vi "4Pi Objective Lock.vi"(7 "Calling VI Ref":refnum<vi>) -> ()   [LabVIEW 2016]
uses:
  Hardware Configuration/Hardware Configuration Controls/Device Type.ctl
  Hardware Configuration/Hardware Configuration Controls/Device Function.ctl
  <vilib>/Utility/miscctls.llb/LVPointTypeDef.ctl
  4Pi Objective Lock Type Defs/4Pi Obj Lock - Actions.ctl
  4Pi Objective Lock Type Defs/4Pi Obj Lock - Notifier Type.ctl
  4Pi Objective Lock Type Defs/4Pi Obj Lock - Lock Settings.ctl
  4Pi Objective Lock Type Defs/4Pi Obj Lock - Camera Settings.ctl
  Device Library/Cameras/Camera Controls/Generic Camera Actions.ctl
  Device Library/Cameras/Camera Controls/Generic Camera ROI.ctl
  <vilib>/addons/control/pid/NI_PID_pid.lvlib
  <vilib>/addons/control/pid/pid.llb/PID (DBL Array).vi
panel:
  in  "Main Tab":T1(tab)
  in  "Update Delay (ms)":i32=10
  in  "D (Derivative)":dbl
  in  "I (Integral)":dbl
  in  "P (Proportional)":dbl=2.0
  in  "Invert Z Axis":bool
  in  "XY Drift Threshold":dbl=0.05
  in  "Abort If Error":bool
  in  "Flip XY Axis":bool
  in  "Invert X Axis":bool
  in  "Invert Y Axis":bool
  in  "Z Stage Move Limit (µm)":dbl=1.0
  in  "Z Drift Threshold":dbl=0.05
  in  "XY Stage Move Limit (µm)":dbl=1.0
  in  "Frame Accumulations":u16=10
  in  "Save Lock Settings":bool
  in  "XY Correction Active":bool=TRUE
  in  "Z Correction Active":bool=TRUE
  in  "Set Camera ROI":bool
  out "Stage Positions":dbl(graph)
  out "Objective Positions":dbl(graph)
  out "X Axis Position (µm)":dbl=1.0
  out "Y Axis Position (µm)":dbl=1.0
  out "Z Axis Position (µm)":dbl=1.0
  out "Measured X Position (px)":dbl=1.0
  out "Measured Y Position (px)":dbl=1.0
  out "Measured Z Position (px)":dbl=1.0
  in  "Start Lock":bool
  out "Error":bool
  in  "Quit":bool
  # "Z Drift Settings"
  # "General Settings"
  # "Camera Setup"
  # "XY Drift Settings"
  # "PID Control Values"
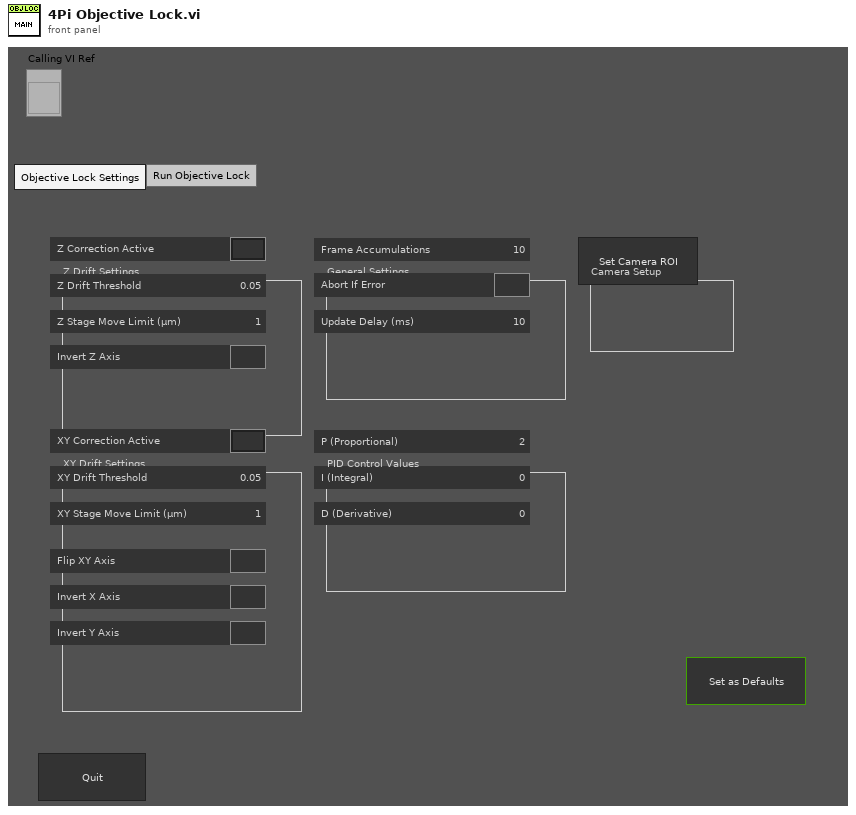
[diagram p1: front panel]
types:
  T1 = enum32{"Objective Lock Settings", "Run Objective Lock"}
  T2 = typedef "4Pi Obj Lock - Camera Settings.ctl" = cluster{"Exposure Time (s)":dbl, "H Offset":u16, "V Offset":u16, "H Width":u16, "V Width":u16}
  T3 = typedef "Device Function.ctl" = enum16{"Primary", "Secondary", "Overview", "Wide Field Drift Correction", "642 nm Excitation", "560 nm Excitation", "546 nm Excitation", "488 nm Excitation", "405 nm Excitation", "Objective Drift Correction", "4Pi Objective Lock", "Objective XY", "Objective Z", "Sample XY", "Sample Coarse Z", "Sample Z", "4Pi Lower", "4Pi Upper", "Adj Cavity", "Line Scanning", "Alert"}
  T4 = typedef "Device Type.ctl" = enum16{"AOTF", "Camera", "Deformable Mirror", "Laser", "Shutter", "Stage", "Waveform", "Email"}
  T5 = typedef "4Pi Obj Lock - Actions.ctl" = enum16{"Idle", "Start Lock", "Get Initial Position", "Get Current Position", "Check Drift", "Move", "Delay", "Abort", "Exit Loop", "Quit"}
  T6 = typedef "4Pi Obj Lock - Lock Settings.ctl" = cluster{"Z Drift Threshold":dbl, "Z Stage Move Limit (µm)":dbl, "XY Drift Threshold":dbl, "XY Stage Move Limit (µm)":dbl, "Frame Accumulations":u16, "Abort If Error":bool, "Flip XY Axis":bool, "Invert X Axis":bool, "Invert Y Axis":bool, "Invert Z Axis":bool, "Z Correction Active":bool, "XY Correction Active":bool, "PID Values":dbl[], "Update Delay (ms)":i32}
  T7 = typedef "4Pi Obj Lock - Notifier Type.ctl" = cluster{"Actions":T5, "Z Drift Threshold":dbl, "Z Stage Move Limit (µm)":dbl, "XY Drift Threshold":dbl, "XY Stage Move Limit (µm)":dbl, "Frame Accumulations":u16, "Abort If Error":bool, "Z Correction Active":bool, "XY Correction Active":bool, "PID Values":dbl[], "Obj Lock Active?":bool, "Update Delay (ms)":i32}
  T8 = enum16{"Always On", "Always Off", "Off While Running"}
  T9 = typedef "LVPointTypeDef.ctl" = cluster{"Horizontal":i16, "Vertical":i16}
  T10 = typedef "Generic Camera Actions.ctl" = enum16{"Status", "Live Preview", "Capture", "Abort", "Set Exposure Time (s)", "Get Exposure Time (s)", "Record Settings", "Set ROI", "Get ROI", "Defect Correction On/Off", "Cooler On/Off", "Fan On/Off", "Quti"}
  T11 = typedef "Generic Camera ROI.ctl" = cluster{"H Offset":u16, "V Offset":u16, "H Width":u16, "V Width":u16}
  T12 = enum32{"Invalid", "Standard", "Closed", "Hidden", "Minimized", "Maximized"}
  T13 = typedef "2D Gaussian - Best Fit Parameters.ctl" = cluster{"Amplitude":dbl, "X Position":dbl, "Y Position":dbl, "X Width":dbl, "Y Width":dbl, "Offset":dbl}
  T14 = cluster{"PID Values[0]":dbl, "PID Values[1]":dbl, "PID Values[2]":dbl}
  T15 = cluster{"PID Values[0]":dbl, "PID Values[1]":dbl, "PID Values[2]":dbl}[]
  T16 = typedef "LVRectTypeDef.ctl" = cluster{"Left":i16, "Top":i16, "Right":i16, "Bottom":i16}
  T17 = typedef "LVBoundsTypeDef.ctl" = cluster{"Width":u32, "Height":u32}
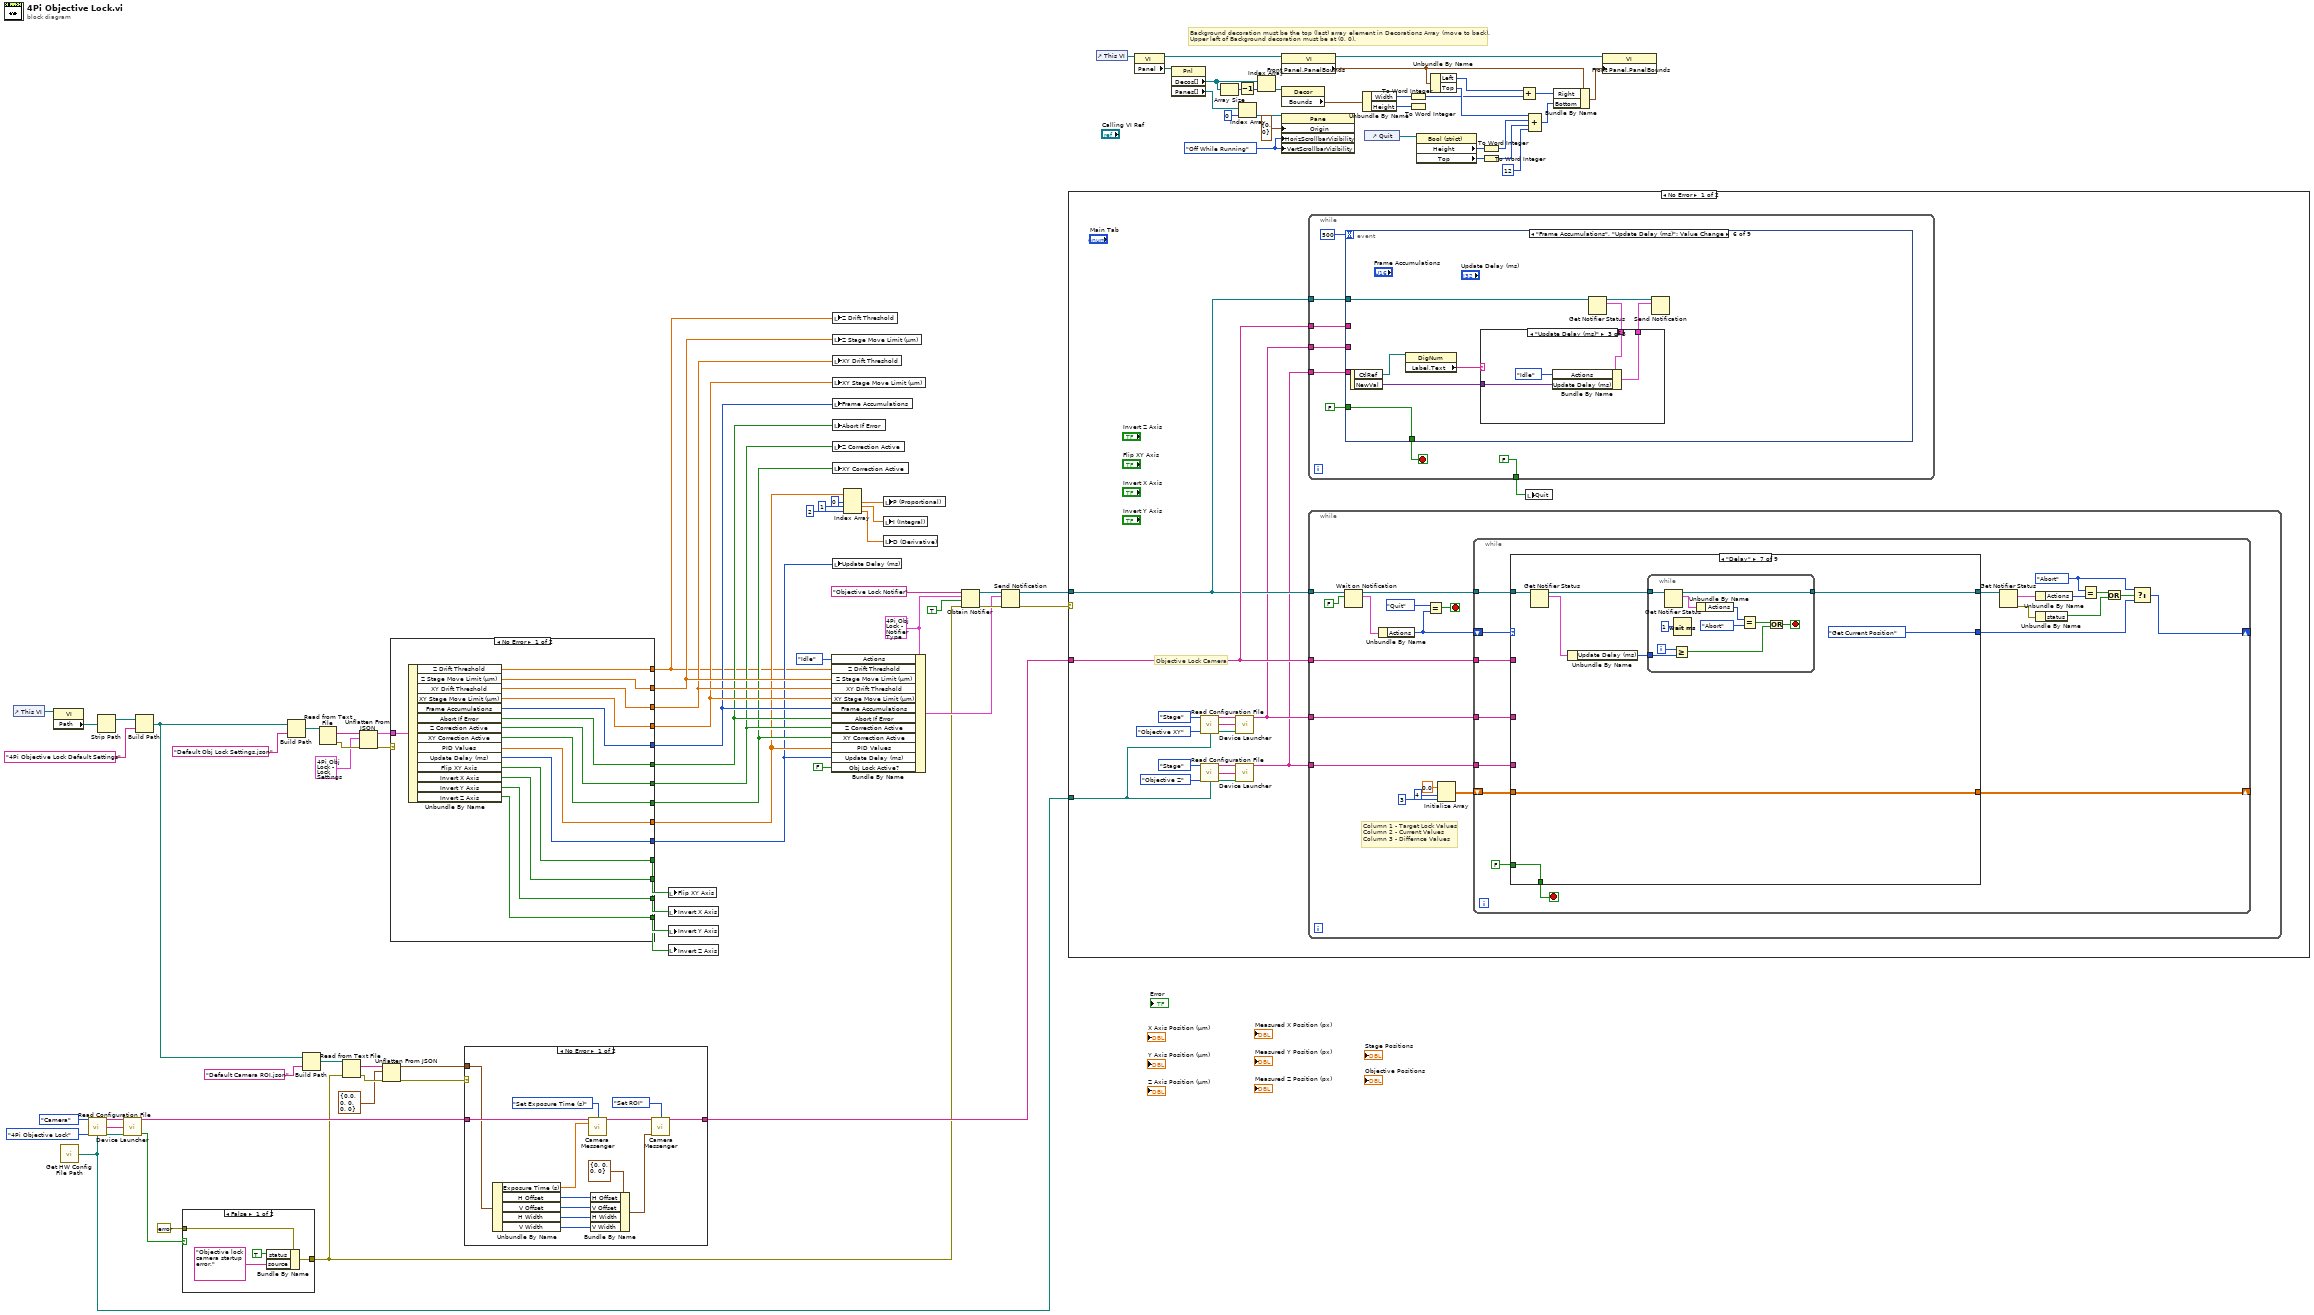
[diagram p0: block diagram]
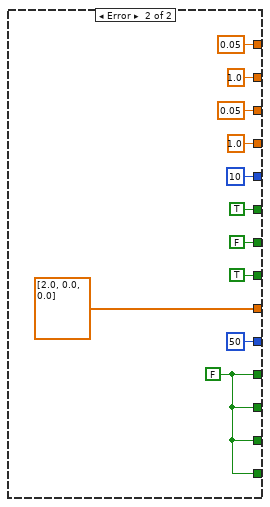
[diagram p4: hidden frame]
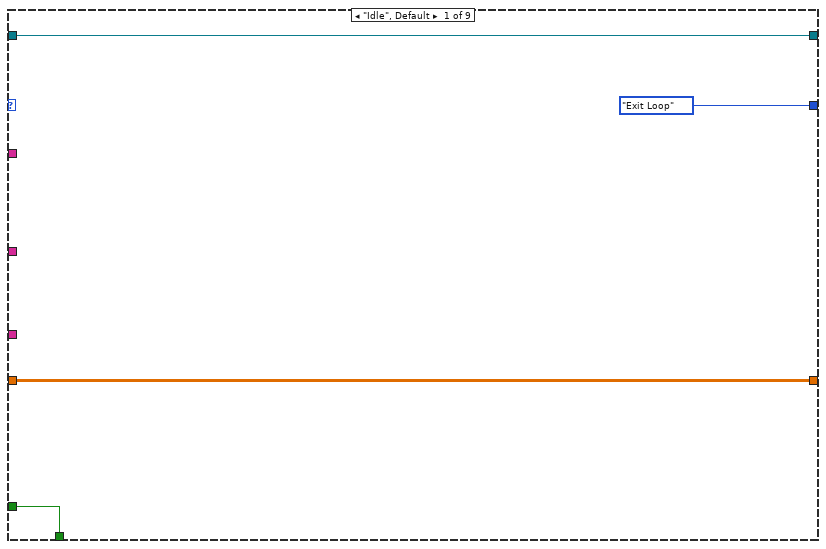
[diagram p5: hidden frame]
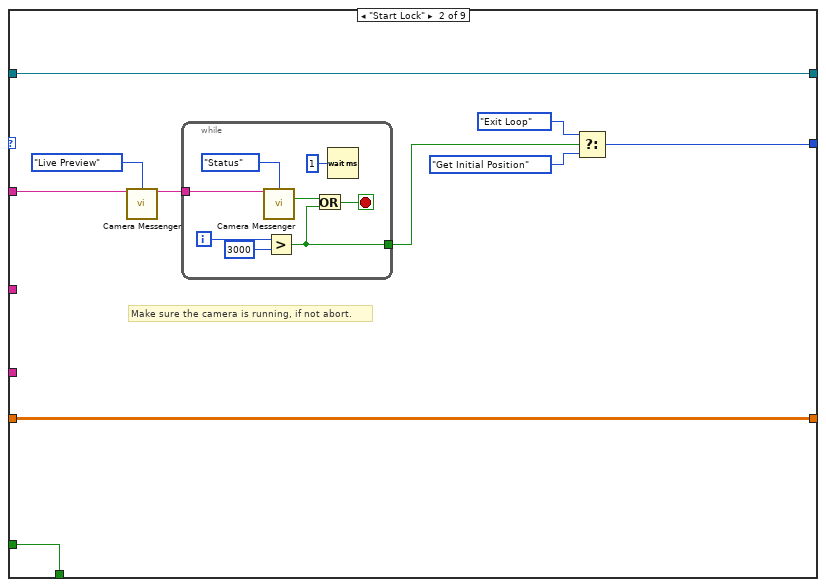
[diagram p6: hidden frame]
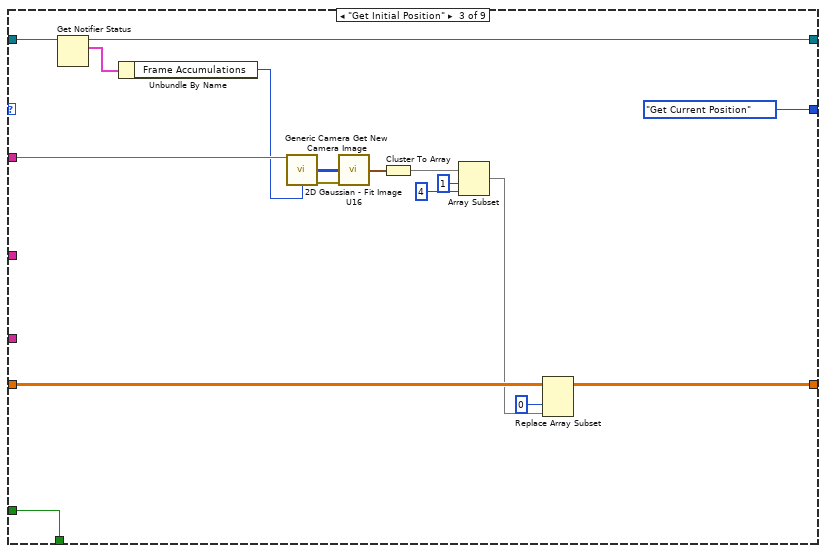
[diagram p7: hidden frame]
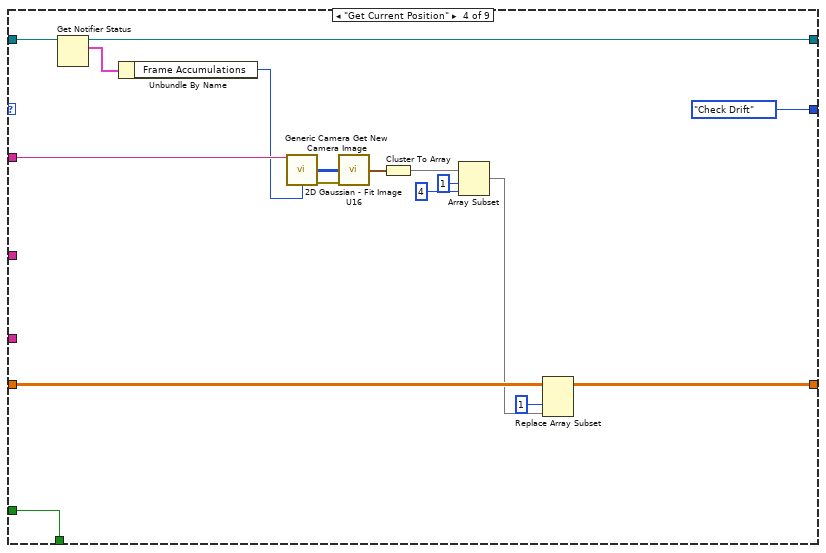
[diagram p8: hidden frame]
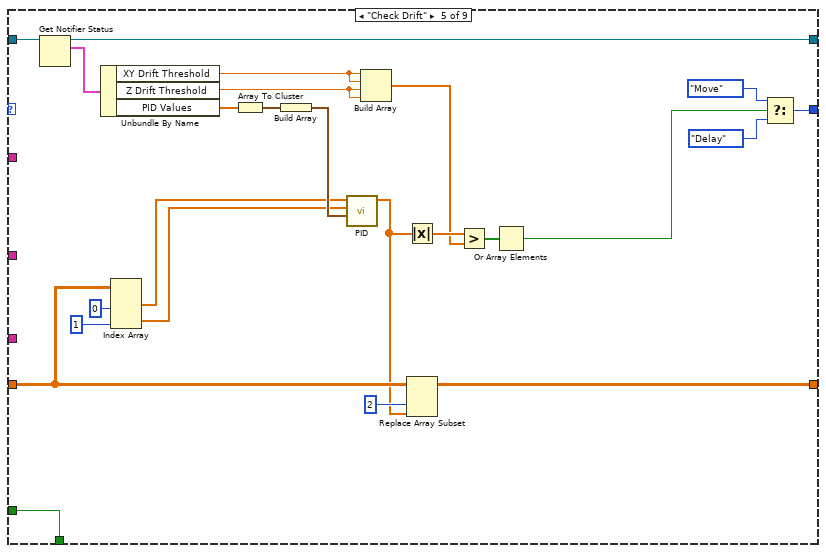
[diagram p9: hidden frame]
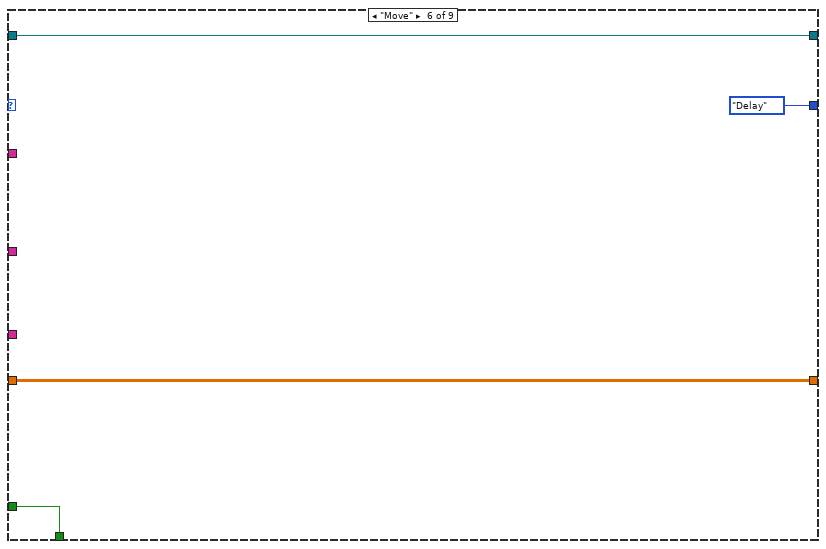
[diagram p10: hidden frame]
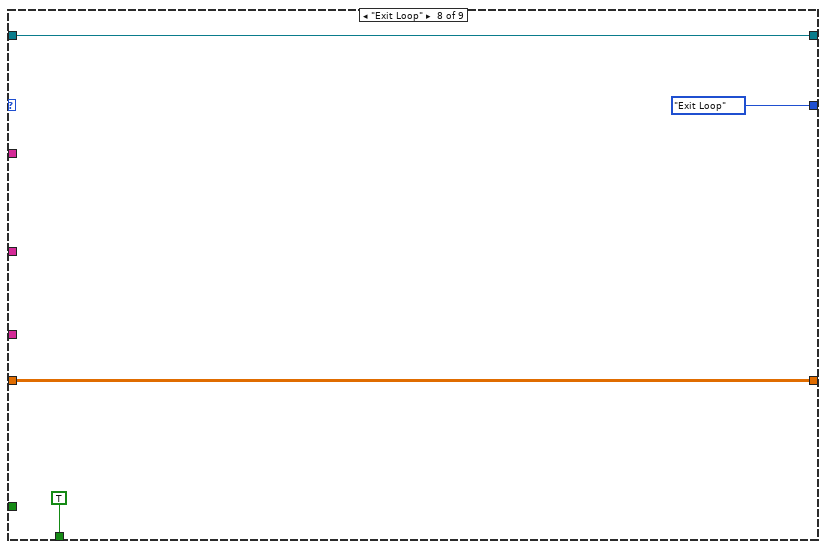
[diagram p11: hidden frame]
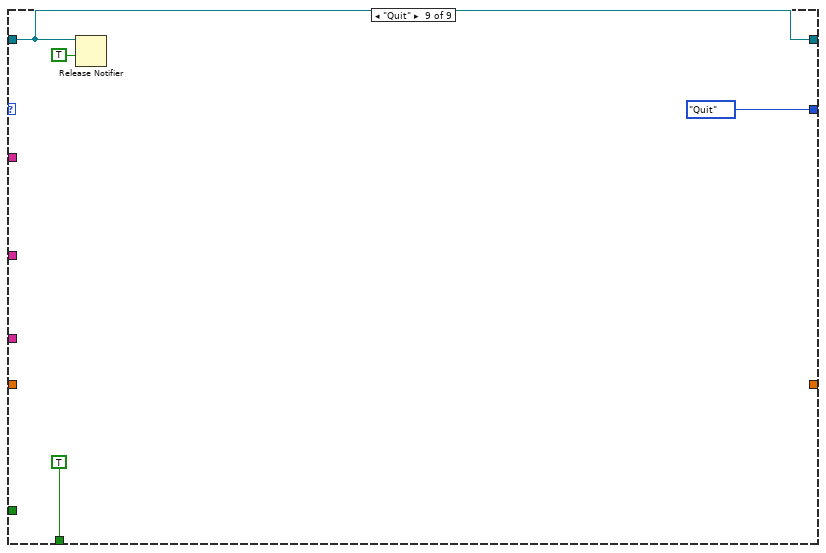
[diagram p12: hidden frame]
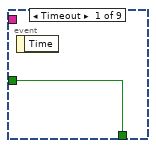
[diagram p13: hidden frame]
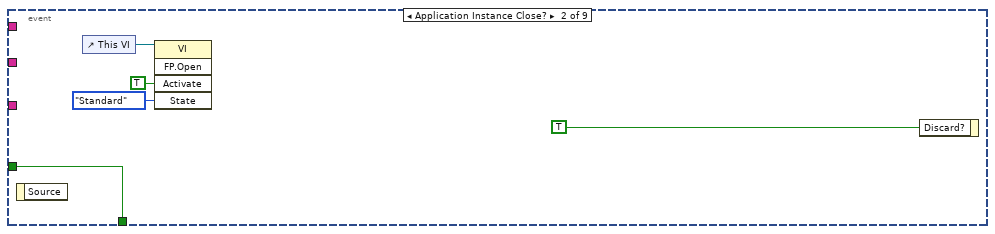
[diagram p14: hidden frame]
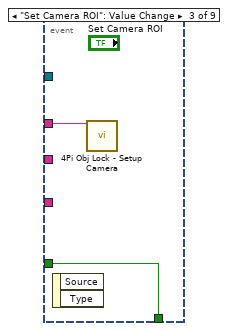
[diagram p15: hidden frame]
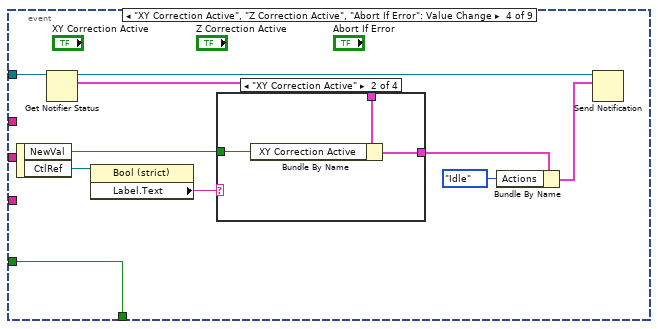
[diagram p16: hidden frame]
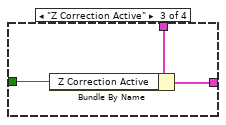
[diagram p18: hidden frame]
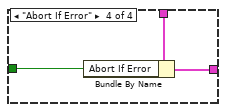
[diagram p19: hidden frame]
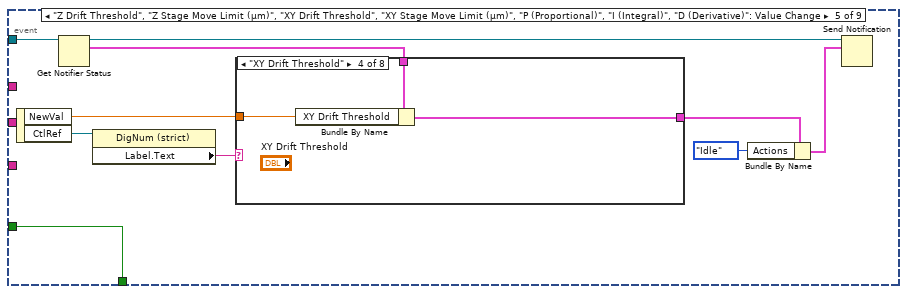
[diagram p20: hidden frame]
diagram:
  w55 = T7 {"Actions"=enum."Idle", "Z Drift Threshold"=0.05, "Z Stage Move Limit (µm)"=1.0, "XY Drift Threshold"=0.05, "XY Stage Move Limit (µm)"=1.0, "Frame Accumulations"=10, "Abort If Error"=FALSE, "Z Correction Active"=FALSE, "XY Correction Active"=FALSE, "PID Values"=[], "Obj Lock Active?"=FALSE, "Update Delay (ms)"=0} ("4Pi Obj Lock")
  w72 = T8."Off While Running" ("Vertical Scrollbar Visibility")
  # "Background decoration must be the top (last) array element in Decorations Array (move to back).\nUpper left of Background decoration must be at (0, 0)."
  n1 = control-ref of="This VI"() -> (w43:refnum<vi>)
  n2 = property class="VI"(reference=w43) -> ("Path"=w24:path)  [unwired: 1 in, 2 out]
  n3 = call "Get HW Config File Path.vi"() -> ("File Path"=w33:path)  [unwired: 14 in, 1 out]
  n4 = call "Read Configuration File.vi"("Device Type"=Device_Type."Camera", "Device Function"=Device_Function."4Pi Objective Lock", "Config File Path"=w33) -> ("Unique Notifier Name"=w40:string, "Device Ports/IDs/Channels"=w42:string[], "Device Engine Path"=w41:path)  [unwired: 9 in, 1 out]
  n5 = Strip Path(path=w24) -> (stripped path=w23:path)  [unwired: 1 out]
  n6 = call "Device Launcher.vi"("Notifier Name"=w40, "Device Ports/IDs/Channels"=w42, "Device Engine Path"=w41) -> ("Notifier Name"=w31:string, "Running?"=w37:bool)  [unwired: 11 in]
  n7 = Build Path(base path=w23, name or relative path="4Pi Objective Lock Default Settings") -> (appended path=w25:path)
  n8 = case shown="False" w37 {
    tunnel: errorcluster {"status"=FALSE, "code"=0, "source"=""} ("Error") -> [w93 w94]
    tunnel: [w90 w94] -> w22
    frame False {
      n9 = Bundle By Name(cluster=w93, "status"=TRUE, "source"="Objective lock camera startup error." ("name or relative path")) -> (w90:errorcluster)
    }
    frame True {
    }
  }
  n10 = Build Path(base path=w25, name or relative path="Default Obj Lock Settings.json") -> (appended path=w52:path)
  n11 = Build Path(base path=w25, name or relative path="Default Camera ROI.json") -> (appended path=w27:path)
  n12 = Read from Text File(file (use dialog)=w52) -> (text=w51:string, error out=w50:errorcluster)  [unwired: 3 in, 2 out]
  n13 = Read from Text File(file (use dialog)=w27, error in=w22) -> (text=w45:string, error out=w44:errorcluster)  [unwired: 2 in, 2 out]
  n14 = Unflatten From JSON(JSON string=w51, type and defaults=T6 {"Z Drift Threshold"=0.05, "Z Stage Move Limit (µm)"=1.0, "XY Drift Threshold"=0.05, "XY Stage Move Limit (µm)"=1.0, "Frame Accumulations"=10, "Abort If Error"=FALSE, "Flip XY Axis"=FALSE, "Invert X Axis"=FALSE, "Invert Y Axis"=FALSE, "Invert Z Axis"=FALSE, "Z Correction Active"=TRUE, "XY Correction Active"=TRUE, "PID Values"=[], "Update Delay (ms)"=0} ("Lock Settings"), error in (no error)=w50) -> (value=w47:T6, error out=w48:errorcluster)  [unwired: 4 in]
  n15 = Unflatten From JSON(JSON string=w45, type and defaults=T2 {"Exposure Time (s)"=0.0, "H Offset"=0, "V Offset"=0, "H Width"=0, "V Width"=0} ("Camera Settings"), error in (no error)=w44) -> (value=w30:T2, error out=w35:errorcluster)  [unwired: 4 in]
  n16 = case shown="No Error" w48 {
    tunnel: [w108 0.05 ("Z Drift Threshold")] -> w1
    tunnel: [w107 1.0 ("Z Stage Move Limit (µm)")] -> w16
    tunnel: [w105 0.05 ("XY Drift Threshold")] -> w15
    tunnel: [w106 1.0 ("XY Stage Move Limit (µm)")] -> w14
    tunnel: [w104 u16 10 ("Frame Accumulations")] -> w13
    tunnel: [w103 TRUE ("Abort If Error")] -> w12
    tunnel: w47 -> [w109 _]
    tunnel: [w102 FALSE ("Z Correction Active")] -> w11
    tunnel: [w101 TRUE ("XY Correction Active")] -> w10
    tunnel: [w100 dbl[] [2.0, 0.0, 0.0] ("PID Values")] -> w9
    tunnel: [w99 u16 50 ("Update Delay (ms)")] -> w2
    tunnel: [w98 w110] -> w18
    tunnel: [w97 w110] -> w19
    tunnel: [w96 w110] -> w20
    tunnel: [w95 w110] -> w21
    frame No Error {
      n17 = Unbundle By Name(w109) -> ("Z Drift Threshold"=w108:dbl, "Z Stage Move Limit (µm)"=w107:dbl, "XY Drift Threshold"=w105:dbl, "XY Stage Move Limit (µm)"=w106:dbl, "Frame Accumulations"=w104:u16, "Abort If Error"=w103:bool, "Z Correction Active"=w102:bool, "XY Correction Active"=w101:bool, "PID Values"=w100:dbl[], "Update Delay (ms)"=w99:i32, "Flip XY Axis"=w95:bool, "Invert X Axis"=w96:bool, "Invert Y Axis"=w97:bool, "Invert Z Axis"=w98:bool)
    }
    frame Error {
      w110 = FALSE ("Flip XY Axis")
    }
  }
  n18 = case shown="No Error" w35 {
    tunnel: w31 -> [w133 w134]
    tunnel: w30 -> [w132 _]
    tunnel: [w124 w134] -> w29
    frame No Error {
      n19 = Unbundle By Name(w132) -> ("Exposure Time (s)"=w126:dbl, "H Offset"=w127:u16, "V Offset"=w128:u16, "H Width"=w129:u16, "V Width"=w130:u16)
      n20 = call "Camera Messenger.vi"("Notifier Name"=w133, "General Camera Actions"=Generic_Camera_Actions."Set Exposure Time (s)", "Exposure Time (s)"=w126) -> ("Notifier Name Dup"=w122:string)  [unwired: 7 in, 5 out]
      n21 = Bundle By Name(cluster=T11 {"H Offset"=0, "V Offset"=0, "H Width"=0, "V Width"=0} ("General Camera ROI"), "H Offset"=w127, "V Offset"=w128, "H Width"=w129, "V Width"=w130) -> (w125:T11)
      n22 = call "Camera Messenger.vi"("Notifier Name"=w122, "General Camera Actions"=Generic_Camera_Actions."Set ROI", "Camera ROI"=w125) -> ("Notifier Name Dup"=w124:string)  [unwired: 7 in, 5 out]
    }
    frame Error {
    }
  }
  n23 = local write "Flip XY Axis"(w21) -> ()
  n24 = local write "Invert X Axis"(w20) -> ()
  n25 = local write "Invert Y Axis"(w19) -> ()
  n26 = local write "Invert Z Axis"(w18) -> ()
  n27 = Bundle By Name(cluster=w55, "Actions"=4Pi_Obj_Lock_-_Actions."Idle", "Z Drift Threshold"=w1, "Z Stage Move Limit (µm)"=w16, "XY Drift Threshold"=w15, "XY Stage Move Limit (µm)"=w14, "Frame Accumulations"=w13, "Abort If Error"=w12, "Z Correction Active"=w11, "XY Correction Active"=w10, "PID Values"=w9, "Update Delay (ms)"=w2, "Obj Lock Active?"=FALSE) -> (w54:T7)
  n28 = local write "Z Drift Threshold"(w1) -> ()
  n29 = local write "Z Stage Move Limit (µm)"(w16) -> ()
  n30 = local write "XY Drift Threshold"(w15) -> ()
  n31 = local write "XY Stage Move Limit (µm)"(w14) -> ()
  n32 = local write "Frame Accumulations"(w13) -> ()
  n33 = local write "Abort If Error"(w12) -> ()
  n34 = local write "Z Correction Active"(w11) -> ()
  n35 = local write "XY Correction Active"(w10) -> ()
  n36 = local write "Update Delay (ms)"(w2) -> ()
  n37 = Index Array(array=w9, index #1=0 ("index"), index #2=1 ("index"), index #3=2 ("index")) -> (element #1=w5:dbl, element #2=w3:dbl, element #3=w4:dbl)
  n38 = local write "P (Proportional)"(w5) -> ()
  n39 = local write "I (Integral)"(w3) -> ()
  n40 = local write "D (Derivative)"(w4) -> ()
  n41 = Obtain Notifier(name (unnamed)="Objective Lock Notifier", notification data type=w55, create if not found? (T)=TRUE, error in (no error)=w22) -> (notifier out=w57:refnum<notifier>, error out=w58:errorcluster)  [unwired: 1 out]
  n42 = Send Notification(notification=w54, notifier=w57, error in (no error)=w58) -> (notifier out=w56:refnum<notifier>, error out=w34:errorcluster)
  n43 = case shown="No Error" w34 {
    tunnel: w33 -> [w139 _]
    tunnel: w56 -> [w137 _]
    tunnel: w29 -> [w138 _]
    frame No Error {
      # "Objective Lock Camera"
      n44 = call "Read Configuration File.vi"("Device Type"=Device_Type."Stage", "Device Function"=Device_Function."Objective XY", "Config File Path"=w139) -> ("Unique Notifier Name"=w147:string, "Device Ports/IDs/Channels"=w145:string[], "Device Engine Path"=w146:path)  [unwired: 9 in, 1 out]
      n45 = call "Read Configuration File.vi"("Device Type"=Device_Type."Stage", "Device Function"=Device_Function."Objective Z", "Config File Path"=w139) -> ("Unique Notifier Name"=w142:string, "Device Ports/IDs/Channels"=w144:string[], "Device Engine Path"=w143:path)  [unwired: 9 in, 1 out]
      n46 = call "Device Launcher.vi"("Notifier Name"=w147, "Device Ports/IDs/Channels"=w145, "Device Engine Path"=w146) -> ("Notifier Name"=w136:string)  [unwired: 11 in, 1 out]
      n47 = call "Device Launcher.vi"("Notifier Name"=w142, "Device Ports/IDs/Channels"=w144, "Device Engine Path"=w143) -> ("Notifier Name"=w135:string)  [unwired: 11 in, 1 out]
      n48 = while {
        tunnel: [FALSE] -> w150
        tunnel: w138 -> [w298]
        tunnel: w137 -> [w297]
        tunnel: w136 -> [w296]
        tunnel: w135 -> [w295]
        stop <- w300 stop-if-true
        n49 = event shown="[5] \"Frame Accumulations\", \"Update Delay (ms)\": Value Change" {
          selector: _ -> [_ _ _ _ _ _ _ _ _]
          dyn-events: _ -> [_ _ _ _ _ _ _ _ _]
          timeout: 500 -> [_ _ _ _ _ _ _ _ _]
          tunnel: FALSE -> [w303 w307 w310 w320 w340 w379 w414 w423 _]
          tunnel: [w303 w307 w310 w320 w340 w379 w414 w423 w433] -> w300
          tunnel: w298 -> [_ _ w309 _ _ _ _ _ _]
          tunnel: w297 -> [_ _ _ w319 w337 w378 w413 w422 w428]
          tunnel: w296 -> [_ _ _ _ _ _ _ _ _]
          tunnel: w295 -> [_ _ _ _ _ _ _ _ _]
          event Timeout {
            n50 = event-data() -> ()  [unwired: 1 in, 1 out]
          }
          event Application Instance Close? {
            n51 = event-data() -> ()  [unwired: 1 in, 1 out]
            n52 = control-ref of="This VI"() -> (w304:refnum<vi>)
            n53 = invoke class="VI" method="FP.Open"(reference=w304, "Activate"=TRUE ("Activate?"), "State"=T12."Standard") -> ()  [unwired: 2 in, 5 out]
            n54 = event-data("Discard?"=TRUE) -> ()  [unwired: 1 in, 1 out]
          }
          event "Set Camera ROI": Value Change {
            n55 = event-data() -> ()  [unwired: 1 in, 2 out]
            n56 = call "4Pi Obj Lock - Setup Camera.vi"("Camera Notifier Name"=w309) -> ()  [unwired: 14 in, 1 out]
          }
          event "XY Correction Active", "Z Correction Active", "Abort If Error": Value Change {
            n57 = event-data() -> ("NewVal"=w315:bool, "CtlRef"=w318:refnum<vi>)  [unwired: 1 in]
            n58 = Get Notifier Status(notifier=w319) -> (notifier out=w317:refnum<notifier>, current notification=w314:T7)  [unwired: 1 in, 3 out]
            n59 = property class="Bool (strict)"(reference=w318) -> ("Label.Text"=w316:string)  [unwired: 1 in, 2 out]
            n60 = case shown="\"XY Correction Active\"" w316 {
              tunnel: w315 -> [_ w323 w326 w329]
              tunnel: w314 -> [w321 w324 w327 w330]
              tunnel: [w321 w322 w325 w328] -> w313
              frame Default {
              }
              frame "XY Correction Active" {
                n61 = Bundle By Name(cluster=w324, "XY Correction Active"=w323) -> (w322:T7)
              }
              frame "Z Correction Active" {
                n62 = Bundle By Name(cluster=w327, "Z Correction Active"=w326) -> (w325:T7)
              }
              frame "Abort If Error" {
                n63 = Bundle By Name(cluster=w330, "Abort If Error"=w329) -> (w328:T7)
              }
            }
            n64 = Bundle By Name(cluster=w313, "Actions"=4Pi_Obj_Lock_-_Actions."Idle") -> (w311:T7)
            n65 = Send Notification(notification=w311, notifier=w317) -> ()  [unwired: 1 in, 2 out]
          }
          event "Z Drift Threshold", "Z Stage Move Limit (µm)", "XY Drift Threshold", "XY Stage Move Limit (µm)", "P (Proportional)", "I (Integral)", "D (Derivative)": Value Change {
            n66 = event-data() -> ("NewVal"=w335:dbl, "CtlRef"=w336:refnum<vi>)  [unwired: 1 in]
            n67 = Get Notifier Status(notifier=w337) -> (notifier out=w334:refnum<notifier>, current notification=w338:T7)  [unwired: 1 in, 3 out]
            n68 = property class="DigNum (strict)"(reference=w336) -> ("Label.Text"=w339:string)  [unwired: 1 in, 2 out]
            n69 = case shown="\"XY Drift Threshold\"" w339 {
              tunnel: w335 -> [_ w343 w346 w349 w352 w357 w363 w369]
              tunnel: w338 -> [w341 w344 w347 w350 w353 w356 w362 w368]
              tunnel: [w341 w342 w345 w348 w351 w354 w360 w366] -> w332
              frame Default {
              }
              frame "Z Drift Threshold" {
                n70 = Bundle By Name(cluster=w344, "Z Drift Threshold"=w343) -> (w342:T7)
              }
              frame "Z Stage Move Limit (µm)" {
                n71 = Bundle By Name(cluster=w347, "Z Stage Move Limit (µm)"=w346) -> (w345:T7)
              }
              frame "XY Drift Threshold" {
                n72 = Bundle By Name(cluster=w350, "XY Drift Threshold"=w349) -> (w348:T7)
              }
              frame "XY Stage Move Limit (µm)" {
                n73 = Bundle By Name(cluster=w353, "XY Stage Move Limit (µm)"=w352) -> (w351:T7)
              }
              frame "P (Proportional)" {
                n74 = Unbundle By Name(w356) -> ("PID Values"=w359:dbl[])
                n75 = Replace Array Subset(array=w359, new element=w357, index=0) -> (w355:dbl[])
                n76 = Bundle By Name(cluster=w356, "PID Values"=w355) -> (w354:T7)
              }
              frame "I (Integral)" {
                n77 = Unbundle By Name(w362) -> ("PID Values"=w365:dbl[])
                n78 = Replace Array Subset(array=w365, new element=w363, index=1) -> (w361:dbl[])
                n79 = Bundle By Name(cluster=w362, "PID Values"=w361) -> (w360:T7)
              }
              frame "D (Derivative)" {
                n80 = Unbundle By Name(w368) -> ("PID Values"=w371:dbl[])
                n81 = Replace Array Subset(array=w371, new element=w369, index=2) -> (w367:dbl[])
                n82 = Bundle By Name(cluster=w368, "PID Values"=w367) -> (w366:T7)
              }
            }
            n83 = Bundle By Name(cluster=w332, "Actions"=4Pi_Obj_Lock_-_Actions."Idle") -> (w331:T7)
            n84 = Send Notification(notification=w331, notifier=w334) -> ()  [unwired: 1 in, 2 out]
          }
          event "Frame Accumulations", "Update Delay (ms)": Value Change {
            n85 = event-data() -> ("CtlRef"=w373:refnum<vi>, "NewVal"=w375:variant)  [unwired: 1 in]
            n86 = property class="DigNum"(reference=w373) -> ("Label.Text"=w372:string)  [unwired: 1 in, 2 out]
            n87 = Get Notifier Status(notifier=w378) -> (notifier out=w377:refnum<notifier>, current notification=w376:T7)  [unwired: 1 in, 3 out]
            n88 = case shown="\"Update Delay (ms)\"" w372 {
              tunnel: w376 -> [w380 w384 w388]
              tunnel: w375 -> [_ w383 w387]
              tunnel: [w380 w381 w385] -> w374
              frame Default {
              }
              frame "Frame Accumulations" {
                n89 = Bundle By Name(cluster=w384, "Actions"=4Pi_Obj_Lock_-_Actions."Idle", "Frame Accumulations"=w383) -> (w381:T7)
              }
              frame "Update Delay (ms)" {
                n90 = Bundle By Name(cluster=w388, "Actions"=4Pi_Obj_Lock_-_Actions."Idle", "Update Delay (ms)"=w387) -> (w385:T7)
              }
            }
            n91 = Send Notification(notification=w374, notifier=w377) -> ()  [unwired: 1 in, 2 out]
          }
          event "Save Lock Settings": Value Change {
            n92 = event-data() -> ()  [unwired: 1 in, 1 out]
            n93 = Wait on Notification(notifier=w413) -> (notification=w411:T7)  [unwired: 3 in, 3 out]
            n94 = Unbundle By Name(w411) -> ("Z Drift Threshold"=w410:dbl, "Z Stage Move Limit (µm)"=w409:dbl, "XY Drift Threshold"=w408:dbl, "XY Stage Move Limit (µm)"=w407:dbl, "Frame Accumulations"=w406:u16, "Abort If Error"=w405:bool, "Z Correction Active"=w404:bool, "XY Correction Active"=w403:bool, "PID Values"=w393:dbl[])
            n95 = local read "Invert X Axis"() -> (w391:bool)
            n96 = local read "Invert Y Axis"() -> (w390:bool)
            n97 = local read "Invert Z Axis"() -> (w389:bool)
            n98 = local read "Flip XY Axis"() -> (w392:bool)
            n99 = Bundle By Name(cluster=T6 {"Z Drift Threshold"=0.05, "Z Stage Move Limit (µm)"=1.0, "XY Drift Threshold"=0.05, "XY Stage Move Limit (µm)"=1.0, "Frame Accumulations"=10, "Abort If Error"=FALSE, "Flip XY Axis"=FALSE, "Invert X Axis"=FALSE, "Invert Y Axis"=FALSE, "Invert Z Axis"=FALSE, "Z Correction Active"=TRUE, "XY Correction Active"=TRUE, "PID Values"=[], "Update Delay (ms)"=0} ("Lock Settings"), "Z Drift Threshold"=w410, "Z Stage Move Limit (µm)"=w409, "XY Drift Threshold"=w408, "XY Stage Move Limit (µm)"=w407, "Frame Accumulations"=w406, "Abort If Error"=w405, "Z Correction Active"=w404, "XY Correction Active"=w403, "PID Values"=w393, "Flip XY Axis"=w392, "Invert X Axis"=w391, "Invert Y Axis"=w390, "Invert Z Axis"=w389) -> (w402:T6)
            n100 = control-ref of="This VI"() -> (w400:refnum<vi>)
            n101 = Flatten To JSON(anything=w402) -> (JSON string=w395:string)  [unwired: 2 in, 1 out]
            n102 = property class="VI"(reference=w400) -> ("Path"=w397:path)  [unwired: 1 in, 2 out]
            n103 = Strip Path(path=w397) -> (stripped path=w396:path)  [unwired: 1 out]
            n104 = Build Path(base path=w396, name or relative path="4Pi Objective Lock Default Settings") -> (appended path=w398:path)
            n105 = Build Path(base path=w398, name or relative path="Default Obj Lock Settings.json") -> (appended path=w394:path)
            n106 = Write to Text File(file (use dialog)=w394, text=w395) -> ()  [unwired: 2 in, 3 out]
          }
          event "Start Lock": Value Change {
            n107 = event-data() -> ("NewVal"=w419:bool)  [unwired: 1 in]
            n108 = Select(t=4Pi_Obj_Lock_-_Actions."Start Lock", s=w419, f=4Pi_Obj_Lock_-_Actions."Abort" ("Actions")) -> (s? t:f=w417:T5)
            n109 = Get Notifier Status(notifier=w422) -> (notifier out=w421:refnum<notifier>, current notification=w420:T7)  [unwired: 1 in, 3 out]
            n110 = Bundle By Name(cluster=w420, "Actions"=w417) -> (w416:T7)
            n111 = Send Notification(notification=w416, notifier=w421) -> ()  [unwired: 1 in, 2 out]
          }
          event "Quit": Value Change {
            # "Turn off the OBJ lock before quiting."
            n112 = event-data() -> ("NewVal"=w433:bool)  [unwired: 1 in]
            n113 = Get Notifier Status(notifier=w428) -> (notifier out=w426:refnum<notifier>, current notification=w424:T7)  [unwired: 1 in, 3 out]
            n114 = Unbundle By Name(w424) -> ("Obj Lock Active?"=w427:bool)
            n115 = case shown="True" w427 {
              tunnel: w426 -> [w434 w438]
              tunnel: [w434 w435] -> w425
              tunnel: w424 -> [_ w440]
              frame False {
              }
              frame True {
                n116 = Bundle By Name(cluster=w440, "Actions"=4Pi_Obj_Lock_-_Actions."Abort") -> (w437:T7)
                n117 = Send Notification(notification=w437, notifier=w438) -> (notifier out=w436:refnum<notifier>)  [unwired: 1 in, 1 out]
                n118 = while {
                  tunnel: w436 -> [w450]
                  tunnel: [w445] -> w435
                  i -> [w444]
                  stop <- w446 stop-if-true
                  n119 = Get Notifier Status(notifier=w450) -> (notifier out=w445:refnum<notifier>, # waiting=w449:i32)  [unwired: 1 in, 3 out]
                  n120 = Greater?(x=w444, y=1500) -> (0:w442:bool)
                  n121 = Less?(x=w449, y=1) -> (x < y?=w447:bool)
                  n122 = Or(x=w447, y=w442) -> (x .or. y?=w446:bool)
                  n123 = Wait (ms)(milliseconds to wait=u32 1) -> ()  [unwired: 1 out]
                }
              }
            }
            n124 = Get Notifier Status(notifier=w425) -> (notifier out=w430:refnum<notifier>, current notification=w432:T7)  [unwired: 1 in, 3 out]
            n125 = Bundle By Name(cluster=w432, "Actions"=4Pi_Obj_Lock_-_Actions."Quit") -> (w429:T7)
            n126 = Send Notification(notification=w429, notifier=w430) -> ()  [unwired: 1 in, 2 out]
          }
        }
      }
      n127 = while {
        tunnel: w138 -> [w164]
        tunnel: w136 -> [w163]
        tunnel: w135 -> [w162]
        tunnel: w137 -> [w161]
        stop <- w157 stop-if-true
        # "Column 1 - Target Lock Values\nColumn 2 - Current Values\nColumn 3 - Differnce Values"
        n128 = Wait on Notification(notifier=w161, ignore previous (F)=FALSE) -> (notifier out=w155:refnum<notifier>, notification=w159:T7)  [unwired: 2 in, 2 out]
        n129 = Unbundle By Name(w159) -> ("Actions"=w156:T5)
        n130 = Equal?(x=4Pi_Obj_Lock_-_Actions."Quit", y=w156) -> (x = y?=w157:bool)
        n131 = Initialize Array(0.0 ("element"), 4 ("dimension size"), 3 ("dimension size")) -> (w152:dbl[][])
        n132 = while {
          shift-right: [w171] -> _
          shift-left: w156 -> [w179]
          tunnel: w164 -> [w183]
          tunnel: w163 -> [w182]
          tunnel: w162 -> [w181]
          tunnel: w155 -> [w177]
          shift-right: [w165] -> _
          shift-left: w152 -> [w166]
          stop <- w178 stop-if-true
          w173 = 4Pi_Obj_Lock_-_Actions."Abort" ("x")
          n133 = case shown="\"Delay\"" w179 {
            tunnel: w183 -> [_ w194 w221 w238 _ _ _ _ _]
            tunnel: w182 -> [_ _ _ _ _ _ _ _ _]
            tunnel: w181 -> [_ _ _ _ _ _ _ _ _]
            tunnel: FALSE -> [w186 w197 w222 w239 w263 w267 w275 _ _]
            tunnel: [4Pi_Obj_Lock_-_Actions."Exit Loop" ("x") w189 4Pi_Obj_Lock_-_Actions."Get Current Position" ("x") 4Pi_Obj_Lock_-_Actions."Check Drift" ("x") w260 4Pi_Obj_Lock_-_Actions."Delay" ("x") 4Pi_Obj_Lock_-_Actions."Get Current Position" ("x") 4Pi_Obj_Lock_-_Actions."Exit Loop" ("x") 4Pi_Obj_Lock_-_Actions."Quit" ("x")] -> w172
            tunnel: [w186 w197 w222 w239 w263 w267 w275 TRUE TRUE] -> w178
            tunnel: w177 -> [w185 w196 w220 w237 w259 w264 w273 w288 w291]
            tunnel: [w185 w196 w219 w236 w258 w264 w269 w288 w291] -> w176
            tunnel: w166 -> [w184 w188 w214 w231 w243 w266 w272 w287 _]
            tunnel: [w184 w188 w213 w230 w240 w266 w272 w287 _] -> w165
            frame "Idle", Default {
            }
            frame "Start Lock" {
              # "Make sure the camera is running, if not abort."
              n134 = call "Camera Messenger.vi"("Notifier Name"=w194, "General Camera Actions"=Generic_Camera_Actions."Live Preview") -> ("Notifier Name Dup"=w193:string)  [unwired: 8 in, 5 out]
              n135 = while {
                tunnel: w193 -> [w204]
                tunnel: [w199] -> w192
                i -> [w203]
                stop <- w200 stop-if-true
                n136 = call "Camera Messenger.vi"("Notifier Name"=w204, "General Camera Actions"=Generic_Camera_Actions."Status") -> ("Running?"=w201:bool)  [unwired: 8 in, 5 out]
                n137 = Greater?(x=w203, y=3000) -> (0:w199:bool)
                n138 = Or(x=w201, y=w199) -> (x .or. y?=w200:bool)
                n139 = Wait (ms)(milliseconds to wait=u32 1) -> ()  [unwired: 1 out]
              }
              n140 = Select(t=4Pi_Obj_Lock_-_Actions."Exit Loop" ("x"), s=w192, f=4Pi_Obj_Lock_-_Actions."Get Initial Position" ("x")) -> (s? t:f=w189:T5)
            }
            frame "Get Initial Position" {
              n141 = Get Notifier Status(notifier=w220) -> (notifier out=w219:refnum<notifier>, current notification=w218:T7)  [unwired: 1 in, 3 out]
              n142 = Unbundle By Name(w218) -> ("Frame Accumulations"=w217:u16)
              n143 = call "Generic Camera Get New Camera Image.vi"("Camera Notifier Name"=w221, "Frames"=w217) -> ("Image - U16"=w216:u16[][], "Error"=w215:errorcluster)  [unwired: 11 in, 1 out]
              n144 = call "2D Gaussian - Fit Image U16.vi"("Image In (U16)"=w216, "Error In"=w215) -> ("Best Fit Params"=w210:T13)  [unwired: 12 in, 1 out]
              n145 = Cluster To Array(cluster=w210) -> (array=w209:dbl[])
              n146 = Array Subset(array=w209, index=1, length=4) -> (w206:dbl[])
              n147 = Replace Array Subset(array=w214, new element=w206, index (col)=0 ("index")) -> (w213:dbl[][])  [unwired: 1 in]
            }
            frame "Get Current Position" {
              n148 = Get Notifier Status(notifier=w237) -> (notifier out=w236:refnum<notifier>, current notification=w235:T7)  [unwired: 1 in, 3 out]
              n149 = Unbundle By Name(w235) -> ("Frame Accumulations"=w234:u16)
              n150 = call "Generic Camera Get New Camera Image.vi"("Camera Notifier Name"=w238, "Frames"=w234) -> ("Image - U16"=w233:u16[][], "Error"=w232:errorcluster)  [unwired: 11 in, 1 out]
              n151 = call "2D Gaussian - Fit Image U16.vi"("Image In (U16)"=w233, "Error In"=w232) -> ("Best Fit Params"=w227:T13)  [unwired: 12 in, 1 out]
              n152 = Cluster To Array(cluster=w227) -> (array=w226:dbl[])
              n153 = Array Subset(array=w226, index=1, length=4) -> (w223:dbl[])
              n154 = Replace Array Subset(array=w231, new element=w223, index (col)=1 ("index")) -> (w230:dbl[][])  [unwired: 1 in]
            }
            frame "Check Drift" {
              n155 = Get Notifier Status(notifier=w259) -> (notifier out=w258:refnum<notifier>, current notification=w257:T7)  [unwired: 1 in, 3 out]
              n156 = Unbundle By Name(w257) -> ("XY Drift Threshold"=w253:dbl, "Z Drift Threshold"=w252:dbl, "PID Values"=w256:dbl[])
              n157 = Index Array(array=w243, index (col) #1=0 ("disabled index (col)"), index (col) #2=1 ("index (col)")) -> (element #1=w245:dbl[], element #2=w244:dbl[])  [unwired: 2 in]
              n158 = Array To Cluster(array=w256) -> (cluster=w255:T14)
              n159 = Build Array(w255) -> (w254:T15)
              n160 = call-poly <vilib>:"PID.vi"("PID gains"=w254, "process variable"=w244, "setpoint"=w245) -> ("output"=w241:dbl[])  [unwired: 7 in, 1 out]
              n161 = Build Array(w253, w253, w252, w252) -> (w250:dbl[])
              n162 = Absolute Value(x=w241) -> (abs(x)=w251:dbl[])
              n163 = Replace Array Subset(array=w243, new element=w241, index (col)=2 ("disabled index (col)")) -> (w240:dbl[][])  [unwired: 1 in]
              n164 = Greater?(x=w251, y=w250) -> (0:w249:bool[])
              n165 = Or Array Elements(Boolean array=w249) -> (logical OR=w248:bool)
              n166 = Select(t=4Pi_Obj_Lock_-_Actions."Move" ("x"), s=w248, f=4Pi_Obj_Lock_-_Actions."Delay" ("x")) -> (s? t:f=w260:T5)
            }
            frame "Move" {
            }
            frame "Delay" {
              n167 = Get Notifier Status(notifier=w273) -> (notifier out=w271:refnum<notifier>, current notification=w274:T7)  [unwired: 1 in, 3 out]
              n168 = Unbundle By Name(w274) -> ("Update Delay (ms)"=w270:i32)
              n169 = while {
                tunnel: w271 -> [w286]
                tunnel: w270 -> [w283]
                tunnel: [w279] -> w269
                i -> [w284]
                stop <- w276 stop-if-true
                n170 = Get Notifier Status(notifier=w286) -> (notifier out=w279:refnum<notifier>, current notification=w282:T7)  [unwired: 1 in, 3 out]
                n171 = Greater Or Equal?(x=w284, y=w283) -> (x >= y?=w277:bool)
                n172 = Wait (ms)(milliseconds to wait=u32 1) -> ()  [unwired: 1 out]
                n173 = Unbundle By Name(w282) -> ("Actions"=w281:T5)
                n174 = Equal?(x=w281, y=4Pi_Obj_Lock_-_Actions."Abort") -> (x = y?=w278:bool)
                n175 = Or(x=w278, y=w277) -> (x .or. y?=w276:bool)
              }
            }
            frame "Exit Loop" {
            }
            frame "Quit" {
              n176 = Release Notifier(notifier=w291, force destroy? (F)=TRUE) -> ()  [unwired: 1 in, 3 out]
            }
          }
          n177 = Get Notifier Status(notifier=w176) -> (current notification=w175:T7, error out=w170:errorcluster)  [unwired: 1 in, 3 out]
          n178 = Unbundle By Name(w175) -> ("Actions"=w174:T5)
          n179 = Unbundle By Name(w170) -> ("status"=w168:bool)
          n180 = Equal?(x=w173, y=w174) -> (x = y?=w169:bool)
          n181 = Or(x=w169, y=w168) -> (x .or. y?=w167:bool)
          n182 = Select(t=w173, s=w167, f=w172) -> (s? t:f=w171:T5)
        }
      }
      n183 = local write "Quit"(w150) -> ()
    }
    frame Error {
    }
  }
  n184 = control-ref of="This VI"() -> (w64:refnum<vi>)
  n185 = property class="VI"(reference=w64) -> (reference out=w73:refnum<vi>, "Panel"=w65:refnum<vi>)  [unwired: 1 in, 1 out]
  n186 = property class="Pnl"(reference=w65) -> ("Decos[]"=w63:refnum<vi>[], "Panes[]"=w69:refnum<vi>[])  [unwired: 1 in, 2 out]
  n187 = Array Size(array=w63) -> (size(s)=w61:i32)
  n188 = Decrement(x=w61) -> (x-1=w62:i32)
  n189 = Index Array(array=w69, index=0) -> (element=w68:refnum<vi>)
  n190 = Index Array(array=w63, index=w62) -> (element=w71:refnum<vi>)
  n191 = property class="VI"(reference=w73) -> (reference out=w75:refnum<vi>, "Front Panel.PanelBounds"=w76:T16)  [unwired: 1 in, 1 out]
  n192 = property class="Decor"(reference=w71) -> ("Bounds"=w74:T17)  [unwired: 1 in, 2 out]
  n193 = property class="Pane"(reference=w68, "Origin"=T9 {"Horizontal"=0, "Vertical"=0}, "HorizScrollbarVisibility"=w72, "VertScrollbarVisibility"=w72) -> ()  [unwired: 1 in, 2 out]
  n194 = Unbundle By Name(w74) -> ("Width"=w79:u32, "Height"=w82:u32)
  n195 = control-ref of="Quit"() -> (w66:refnum<vi>)
  n196 = To Word Integer(number=w79) -> (16bit integer=w81:i16)
  n197 = To Word Integer(number=w82) -> ()  [unwired: 1 out]
  n198 = property class="Bool (strict)"(reference=w66) -> ("Height"=w84:u32, "Top"=w85:i32)  [unwired: 1 in, 2 out]
  n199 = Unbundle By Name(w76) -> ("Left"=w78:i16, "Top"=w89:i16)
  n200 = To Word Integer(number=w84) -> (16bit integer=w87:i16)
  n201 = To Word Integer(number=w85) -> (16bit integer=w88:i16)
  n202 = Add(x=w78, y=w81) -> (x+y=w80:i16)
  n203 = Compound Arithmetic op=ADD(w89, w87, w88, i16 12 ("y")) -> (w83:i16)
  n204 = Bundle By Name(cluster=w76, "Right"=w80, "Bottom"=w83) -> (w77:T16)
  n205 = property class="VI"(reference=w75, "Front Panel.PanelBounds"=w77) -> ()  [unwired: 1 in, 2 out]
